vi "Event_ball_out_of_vision.vi"(8 "error in (no error)":errorcluster, 10 "Game in":refnum<class "Game.lvclass">, 11 "Events in":refnum<class "Events.lvclass">) -> (0 "error out":errorcluster, 3 "Events out":refnum<class "Events.lvclass">)   [LabVIEW 2018, in "Events.lvclass"]
uses:
  Events.lvclass
  Game_class/Game.lvclass
  Game_class/Game.lvclass/Game.ctl
  Ball_class/Ball.lvclass/Ball.ctl
  Events.lvclass/Events.ctl
  Game_class/Read BallRef.vi
  Ball_class/Read Valid.vi
  Write ball_out_of_vision.vi
  Ball_class/Ball.lvclass
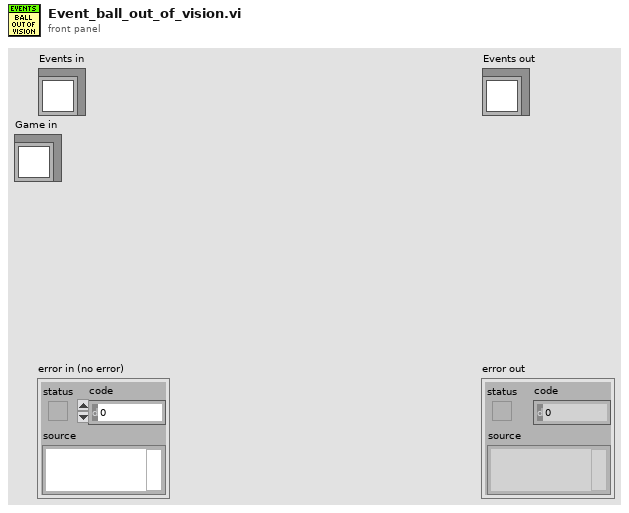
[diagram p1: front panel]
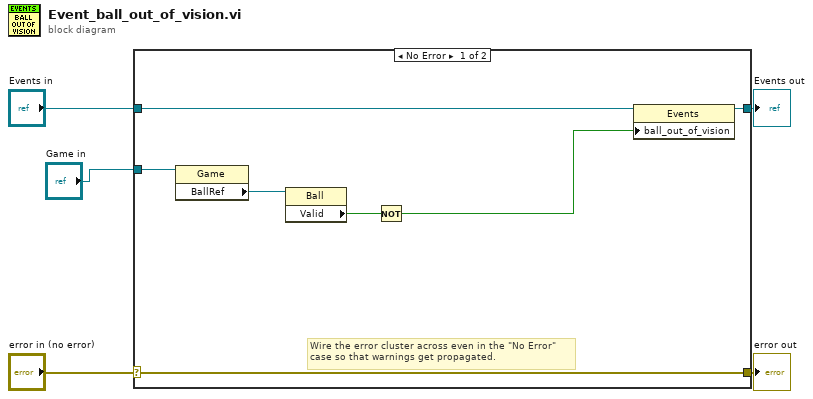
[diagram p0: block diagram]
diagram:
  n1 = case shown="No Error" "error in (no error)" {
    selector: "error in (no error)" -> [w12 w14]
    tunnel: [w12 w14] -> w4
    tunnel: [w10 w13] -> w2
    tunnel: "Events in" -> [w11 w13]
    tunnel: "Game in" -> [w9 _]
    frame No Error {
      # "Wire the error cluster across even in the \"No Error\"\ncase so that warnings get propagated."
      n2 = property class="Game"(reference=w9) -> ("BallRef"=w8:refnum<class "Ball.lvclass">)  [unwired: 1 in, 2 out]
      n3 = property class="Ball"(reference=w8) -> ("Valid"=w7:bool)  [unwired: 1 in, 2 out]
      n4 = Not(x=w7) -> (.not. x?=w6:bool)
      n5 = property class="Events"(reference=w11, "ball_out_of_vision"=w6) -> (reference out=w10:refnum<class "Events.lvclass">)  [unwired: 1 in, 1 out]
    }
    frame Error {
    }
  }
  "error out" <- w4
  "Events out" <- w2
